vi "Set Counting Mode.vi"(8 "error in (no error)":errorcluster, 10 "Mode (def: A,B for T preset)":T1, 11 "VISA resource name":refnum<visa-resource-name>) -> (0 "error out":errorcluster, 3 "VISA resource name out":refnum<visa-resource-name>)   [LabVIEW 2023, in "SR400.lvlib"]
uses:
  SR400.lvlib
  Typedefs.llb/Counter Mode.ctl
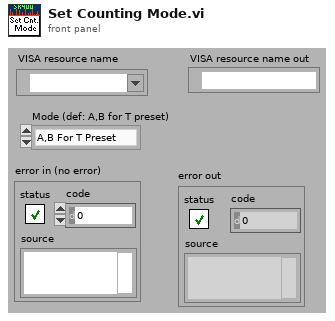
[diagram p1: front panel]
types:
  T1 = typedef "SR400.lvlib/Counter Mode.ctl" = enum16{"A,B For T Preset", "A-B For T Preset", "A+B For T Preset", "A For B Preset"}
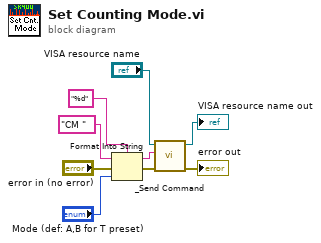
[diagram p0: block diagram]
diagram:
  n1 = Format Into String(format string="%d", initial string="CM " ("command"), error in="error in (no error)", "Mode (def: A,B for T preset)") -> (resulting string=w4:string, error out=w3:errorcluster)
  n2 = call "_Send Command.vi"("error in (no error)"=w3, "Command"=w4, "VISA resource name"="VISA resource name") -> ("error out"=→"error out":errorcluster, "VISA resource name out"=→"VISA resource name out":refnum<visa-resource-name>)  [unwired: 1 in, 6 out]
